vi "FromRepo.vi"(8 "error in":errorcluster, 9 "from repo cluster":T2, 10 "repository in":refnum<class "NISE_CEF_Repository.lvclass">, 11 "group in":refnum<class "Group.lvclass">) -> (0 "error out":errorcluster, 2 "repository out":refnum<class "NISE_CEF_Repository.lvclass">, 3 "root":T1)   [LabVIEW 2013, in "Group.lvclass"]
uses:
  Group.lvclass
  Configuration Framework/Repository/NISE_CEF_Repository.lvclass
  Configuration Framework/Node/FromRepoCluster.ctl
  Configuration Framework/Node/NodeRef.ctl
  Configuration Framework/Node/NISE_CEF_Node.lvclass
  cRIO Repo/cRIORepo.lvclass
  cRIO Repo/cRIORepo.lvclass/cRIORepo.ctl
  Group.lvclass/Group.ctl
  cRIO Repo/Read Channels.vi
  Write GroupName.vi
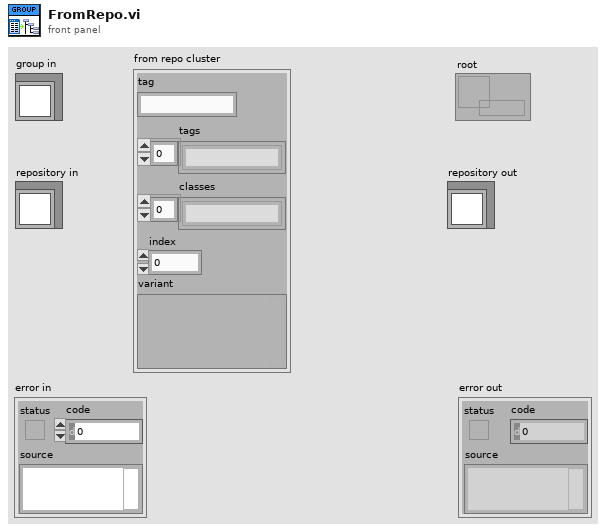
[diagram p1: front panel]
types:
  T1 = typedef "NISE_CEF_Node.lvclass/NodeRef.ctl" = refnum<data-value>
  T2 = typedef "NISE_CEF_Node.lvclass/FromRepoCluster.ctl" = cluster{"tag":string, "tags":string[], "classes":string[], "index":i32, "variant":variant}
  T3 = typedef "Channel.ctl" = cluster{"channel group":string, "channel name":string, "IO ":string, "sensor ID":string, "description":string, "system":string, "channel type":string}
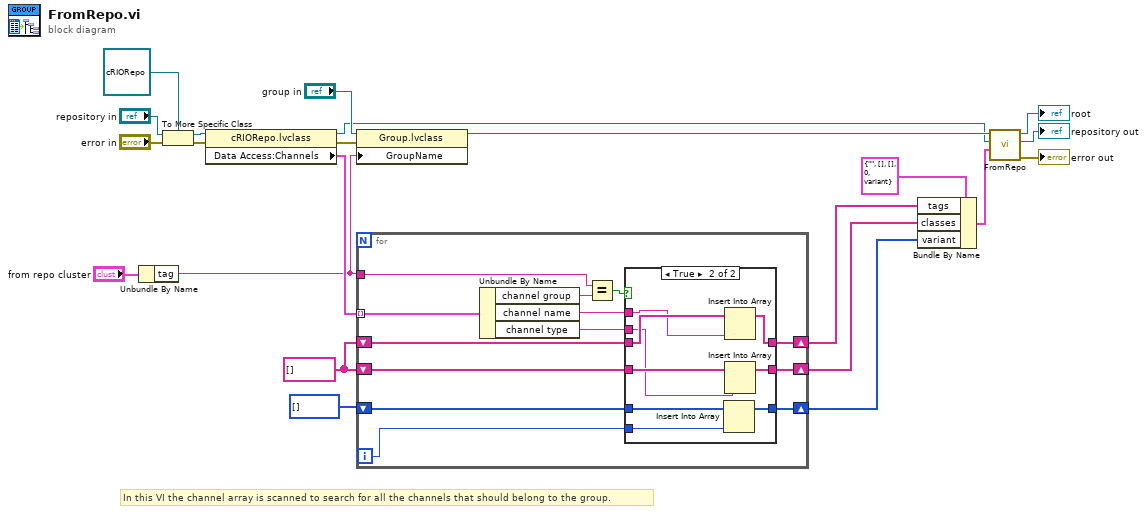
[diagram p0: block diagram]
diagram:
  w9 = string[] [] ("array in")
  # "In this VI the channel array is scanned to search for all the channels that should belong to the group."
  n1 = Unbundle By Name("from repo cluster") -> ("tag"=w3:string)
  n2 = To More Specific Class(target class=refnum<class "cRIORepo.lvclass"> refnum ("cRIO repo.lvclass"), reference="repository in", error in="error in") -> (specific class reference=w20:refnum<class "cRIORepo.lvclass">, error out=w18:errorcluster)
  n3 = property class="cRIORepo.lvclass"(reference=w20, error in=w18) -> (reference out=w5:refnum<class "cRIORepo.lvclass">, error out=w17:errorcluster, "Data Access:Channels"=w19:T3[])
  n4 = property class="Group.lvclass"(reference="group in", error in=w17, "GroupName"=w3) -> (reference out=w6:refnum<class "Group.lvclass">)  [unwired: 1 out]
  n5 = for {
    shift-right: [w33] -> w15
    shift-left: w9 -> [w34]
    tunnel: w19 -> [w35] mode=indexing
    shift-right: [w27] -> w8
    shift-left: w9 -> [w29]
    tunnel: w3 -> [w26]
    shift-right: [w23] -> w1
    shift-left: i32[] [] -> [w25]
    i -> [w24]
    n6 = Unbundle By Name(w35) -> ("channel group"=w31:string, "channel name"=w32:string, "channel type"=w28:string)
    n7 = Equal?(x=w26, y=w31) -> (x = y?=w30:bool)
    n8 = case shown="True" w30 {
      tunnel: w34 -> [w38 w47]
      tunnel: [w38 w46] -> w33
      tunnel: w32 -> [_ w39]
      tunnel: w29 -> [w37 w45]
      tunnel: w28 -> [_ w44]
      tunnel: [w37 w43] -> w27
      tunnel: w25 -> [w36 w42]
      tunnel: w24 -> [_ w40]
      tunnel: [w36 w41] -> w23
      frame False {
      }
      frame True {
        n9 = Insert Into Array(array=w42, new element=w40) -> (w41:i32[])  [unwired: 1 in]
        n10 = Insert Into Array(array=w47, new element=w39) -> (w46:string[])  [unwired: 1 in]
        n11 = Insert Into Array(array=w45, new element=w44) -> (w43:string[])  [unwired: 1 in]
      }
    }
  }
  n12 = Bundle By Name(cluster=T2 {"tag"="", "tags"=[], "classes"=[], "index"=0, "variant"=variant} ("Cluster"), "tags"=w15, "classes"=w8, "variant"=w1) -> (w7:T2)
  n13 = call-parent "FromRepo.vi"("from repo cluster"=w7, "repository in"=w5, "node in"=w6) -> ("error out"=→"error out":errorcluster, "repository out"=→"repository out":refnum<class "NISE_CEF_Repository.lvclass">, "node"=→"root":T1)  [unwired: 6 in]
